vi "subGetItemInfosFromProjectRef.vi"(11 "SolutionBuilder in":refnum<class "SolutionBuilder.lvclass">) -> (3 "SolutionBuilder out":refnum<class "SolutionBuilder.lvclass">)   [LabVIEW 2020, in "SolutionBuilder.lvlib" / "SolutionBuilder.lvclass"]
uses:
  SolutionBuilder.lvclass
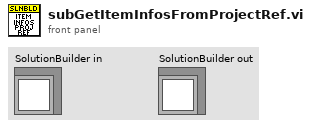
[diagram p1: front panel]
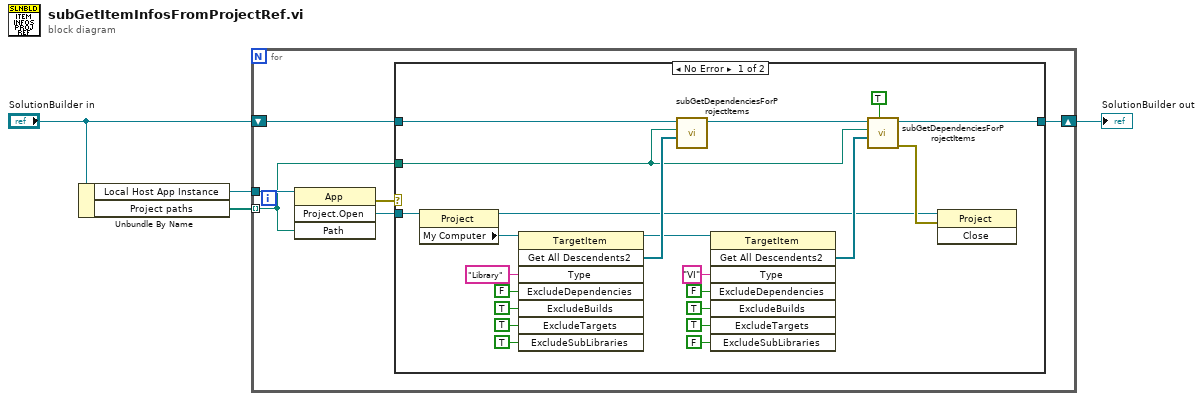
[diagram p0: block diagram]
diagram:
  n1 = Unbundle By Name("SolutionBuilder in") -> ("Local Host App Instance"=w4:refnum<vi>, "Project paths"=w3:path[])
  n2 = for {
    tunnel: w3 -> [w8] mode=indexing
    tunnel: w4 -> [w10]
    shift-right: [w7] -> w1
    shift-left: "SolutionBuilder in" -> [w9]
    n3 = invoke class="App" method="Project.Open"(reference=w10, "Path"=w8) -> (error out=w5:errorcluster, "Project:Open"=w6:refnum<vi>)  [unwired: 2 in, 2 out]
    n4 = case shown="No Error" w5 {
      tunnel: w9 -> [w21 w33]
      tunnel: w8 -> [w17 _]
      tunnel: [w15 w33] -> w7
      tunnel: w6 -> [w12 _]
      frame No Error {
        n5 = property class="Project"(reference=w12) -> (reference out=w11:refnum<vi>, "My Computer"=w22:refnum<vi>)  [unwired: 1 in, 1 out]
        n6 = invoke class="TargetItem" method="Get All Descendents2"(reference=w22, "Type"="Library", "ExcludeDependencies"=FALSE, "ExcludeBuilds"=TRUE, "ExcludeTargets"=TRUE, "ExcludeSubLibraries"=TRUE) -> (reference out=w14:refnum<vi>, "Get All Descendents2"=w20:refnum<vi>[])  [unwired: 2 in, 6 out]
        n7 = call "subGetDependenciesForProjectItems.vi"("Dependents"=w20, "Owning project"=w17, "SolutionBuilder in"=w21) -> ("SolutionBuilder out"=w19:refnum<class "SolutionBuilder.lvclass">)  [unwired: 7 in, 1 out]
        n8 = invoke class="TargetItem" method="Get All Descendents2"(reference=w14, "Type"="VI", "ExcludeDependencies"=FALSE, "ExcludeBuilds"=TRUE, "ExcludeTargets"=TRUE, "ExcludeSubLibraries"=FALSE) -> ("Get All Descendents2"=w16:refnum<vi>[])  [unwired: 2 in, 7 out]
        n9 = call "subGetDependenciesForProjectItems.vi"("Shallow check"=TRUE, "Dependents"=w16, "Owning project"=w17, "SolutionBuilder in"=w19) -> ("error out"=w13:errorcluster, "SolutionBuilder out"=w15:refnum<class "SolutionBuilder.lvclass">)  [unwired: 6 in]
        n10 = invoke class="Project" method="Close"(reference=w11, error in=w13) -> ()  [unwired: 1 in, 3 out]
      }
      frame Error {
      }
    }
  }
  "SolutionBuilder out" <- w1
